vi "LS4 SetPitches.vi"(8 "error in (no error)":errorcluster, 11 "DelayLineLS4 in":refnum<class "DLLS4.lvclass">) -> (0 "error out":errorcluster, 3 "DelayLineLS4 out":refnum<class "DLLS4.lvclass">)   [LabVIEW 2015, in "DLLS4.lvclass"]
uses:
  DLLS4.lvclass
  LS4_parameters.ctl
  DelayLine.lvclass/DelayLine.ctl
  GeneralFunctionality/GeneralFunctionality.lvclass/GeneralFunctionality.ctl
  <vilib>/Utility/error.llb/DialogType.ctl
  Config/Config.lvclass
  <vilib>/ErrorRing/Error Ring.xnode
  DelayLine.lvclass
  GeneralFunctionality/GeneralFunctionality.lvclass
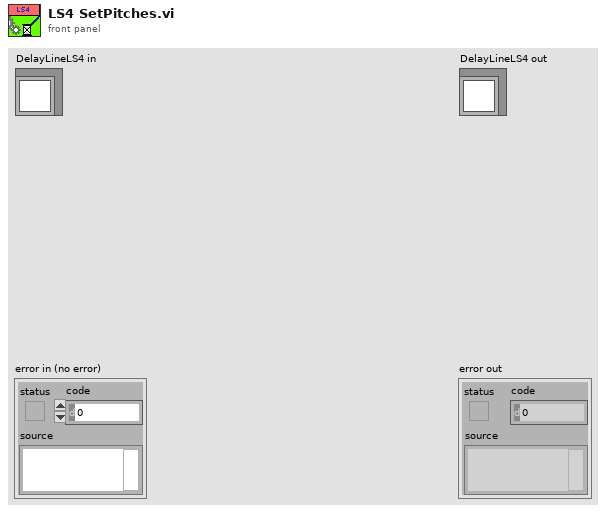
[diagram p1: front panel]
types:
  T1 = typedef "DelayLine.lvclass/LS4_parameters.ctl" = string
  T2 = typedef "DialogType.ctl" = u16
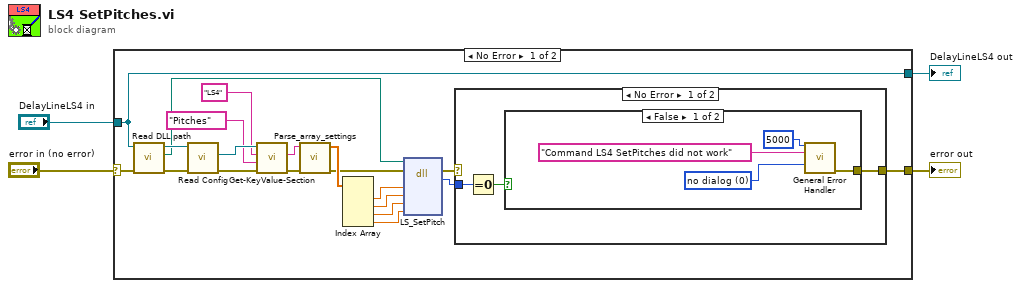
[diagram p0: block diagram]
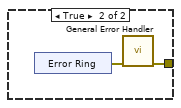
[diagram p2: hidden frame]
diagram:
  n1 = case shown="No Error" "error in (no error)" {
    selector: "error in (no error)" -> [w14 w37]
    tunnel: [w18 w37] -> w3
    tunnel: [w13 w36] -> w1
    tunnel: "DelayLineLS4 in" -> [w13 w36]
    frame No Error {
      n2 = call "Read DLL path.vi"("error in (no error)"=w14, "DelayLine in"=w13) -> ("error out"=w17:errorcluster, "DLL path"=w15:path, "DelayLine out"=w16:refnum<class "DLLS4.lvclass">)  [unwired: 7 in]
      n3 = call "Read Config.vi"("error in (no error)"=w17, "GeneralFunctionality en entrée"=w16) -> ("error out"=w6:errorcluster, "Config.lvclass"=w12:refnum<class "Config.lvclass">)  [unwired: 7 in, 1 out]
      n4 = call-dynamic "Get-KeyValue-Section.vi"("error in (no error)"=w6, "Key"=T1 "Pitches" ("Section"), "Section"="LS4", "Config in"=w12) -> ("error out"=w11:errorcluster, "Value"=w9:string)  [unwired: 5 in, 1 out]
      n5 = call "Parse_array_settings.vi"("error in (no error)"=w11, "Value"=w9) -> ("error out"=w7:errorcluster, "Array"=w8:sgl[])  [unwired: 8 in]
      n6 = Index Array(array=w8) -> (element #1=w21:sgl, element #2=w22:sgl, element #3=w23:sgl, element #4=w24:sgl)  [unwired: 4 in]
      n7 = dll-call lib="S:/TRANCON/DLL/LStep4.dll" fn="LS_SetPitch"(path in=w15, error in=w7, "X"=w21, "Y"=w22, "Z"=w23, "A"=w24) -> (error out=w20:errorcluster, "type de retour"=w19:i32)  [unwired: 5 in, 1 out]
      n8 = case shown="No Error" w20 {
        selector: w20 -> [_ w35]
        tunnel: w19 -> [w27 _]
        tunnel: [w26 w35] -> w18
        frame No Error {
          n9 = Equal To 0?(x=w27) -> (x = 0?=w25:bool)
          n10 = case shown="False" w25 {
            tunnel: [w29 w32] -> w26
            frame False {
              w28 = T2 0 items=["no dialog", "OK message", "continue or stop message", "OK message + warnings", "continue/stop + warnings"] ("type of dialog (OK msg:1)")
              n11 = call <vilib>:"General Error Handler.vi"("[error code] (0)"=5000 ("code"), "[error source] (\" \")"="Command LS4 SetPitches did not work" ("String to Prepend to source (\"\")"), "type of dialog (OK msg:1)"=w28) -> ("error out"=w29:errorcluster)  [unwired: 8 in, 4 out]
            }
            frame True {
              n12 = xnode "Error Ring"() -> ("error out"=w33:errorcluster)
              n13 = call <vilib>:"General Error Handler.vi"("error in (no error)"=w33) -> ("error out"=w32:errorcluster)  [unwired: 10 in, 4 out]
            }
          }
        }
        frame Error {
        }
      }
    }
    frame Error {
    }
  }
  "error out" <- w3
  "DelayLineLS4 out" <- w1
